vi "Write Log Folder.vi"(8 "error in (no error)":errorcluster, 10 "Log Folder":path, 11 "Robot Event Local Log in":refnum<class "Robot Event Local Log.lvclass">) -> (0 "error out":errorcluster, 3 "Robot Event Local Log out":refnum<class "Robot Event Local Log.lvclass">)   [LabVIEW 2019, in "Robot Event Local Log.lvclass"]
uses:
  Robot Event Local Log.lvclass
  Robot Event Local Log.lvclass/Robot Event Local Log.ctl
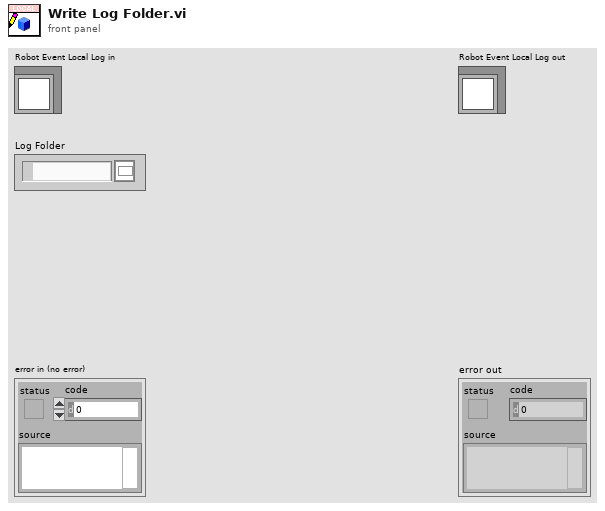
[diagram p1: front panel]
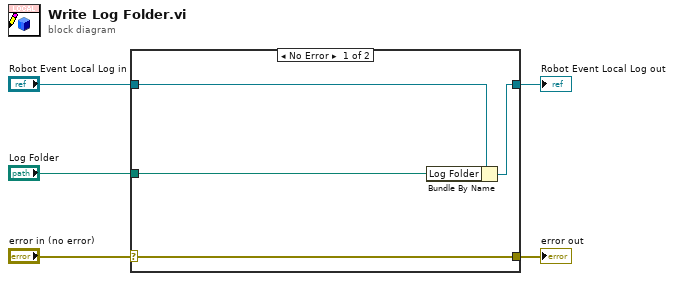
[diagram p0: block diagram]
diagram:
  n1 = case shown="No Error" "error in (no error)" {
    selector: "error in (no error)" -> [w9 w10]
    tunnel: [w9 w10] -> w4
    tunnel: [w7 w11] -> w2
    tunnel: "Robot Event Local Log in" -> [w8 w11]
    tunnel: "Log Folder" -> [w6 _]
    frame No Error {
      n2 = Bundle By Name(cluster=w8, "Log Folder"=w6) -> (w7:refnum<class "Robot Event Local Log.lvclass">)
    }
    frame Error {
    }
  }
  "error out" <- w4
  "Robot Event Local Log out" <- w2
